vi "CSDB_Transfer.get instance data.vi"(0 "connection reference":T1, 1 "InstanceName":string, 2 "error in (no error)":errorcluster) -> (3 "connection reference out":T1, 4 "InstanceName      Classname":string[](array[string]), 5 "InstanceName      AttributeName      Value":string[][](array[string]), 6 "error out":errorcluster)   [LabVIEW 2014, in "CSDB_Transfer.lvlib"]
uses:
  CSDB_Transfer.lvlib
  <vilib>/addons/database/Connection.llb/Conn ObjectReference.ctl
  <vilib>/addons/database/NI_Database_API.lvlib
  CSDB_Common/CSDB_Common.lvlib
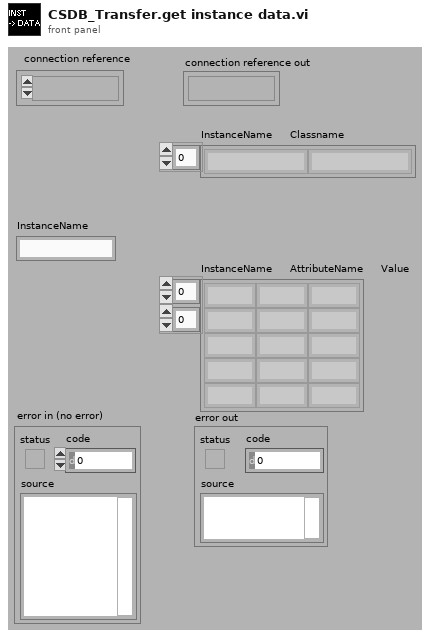
[diagram p1: front panel]
types:
  T1 = typedef "NI_Database_API.lvlib/Conn ObjectReference.ctl" = refnum<k1>
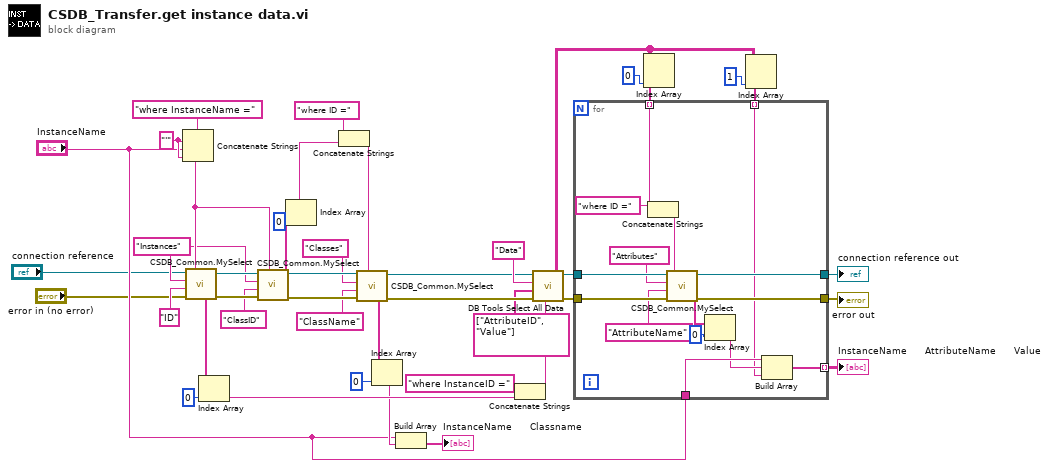
[diagram p0: block diagram]
diagram:
  w37 = "Instances" ("table")
  w42 = "'"
  n1 = Concatenate Strings("where InstanceName =", w42, "InstanceName", w42) -> (w40:string)
  n2 = call "CSDB_Common.MySelect.vi"("optional clause"=w40, "error in (no error)"="error in (no error)", "column"="ID", "table"=w37, "connection reference"="connection reference") -> ("error out"=w38:errorcluster, "1d output array"=w35:string[], "connection reference out"=w39:T1)  [unwired: 2 in]
  n3 = Index Array(array=w35, index=0) -> (element=w15:string)
  n4 = call "CSDB_Common.MySelect.vi"("optional clause"=w40, "error in (no error)"=w38, "column"="ClassID", "table"=w37, "connection reference"=w39) -> ("error out"=w33:errorcluster, "1d output array"=w30:string[], "connection reference out"=w34:T1)  [unwired: 2 in]
  n5 = Index Array(array=w30, index=0) -> (element=w14:string)
  n6 = Concatenate Strings("where ID =", w14) -> (w27:string)
  n7 = call "CSDB_Common.MySelect.vi"("optional clause"=w27, "error in (no error)"=w33, "column"="ClassName", "table"="Classes", "connection reference"=w34) -> ("error out"=w26:errorcluster, "1d output array"=w20:string[], "connection reference out"=w16:T1)  [unwired: 2 in]
  n8 = Index Array(array=w20, index=0) -> (element=w8:string)
  n9 = Build Array("InstanceName", w8) -> (→"InstanceName      Classname":string[])
  n10 = Concatenate Strings("where InstanceID =" ("string"), w15) -> (w22:string)
  n11 = call <vilib>:"DB Tools Select All Data.vi"("optional clause"=w22, "error in (no error)"=w26, "columns"=string[] ["AttributeID", "Value"], "table"="Data", "connection reference"=w16) -> ("error out"=w17:errorcluster, "data"=w13:string[][], "connection reference out"=w18:T1)  [unwired: 1 in]
  n12 = Index Array(array=w13, index (col)=0 ("index")) -> (element=w12:string[])  [unwired: 1 in]
  n13 = Index Array(array=w13, index (col)=1 ("index")) -> (element=w9:string[])  [unwired: 1 in]
  n14 = for {
    tunnel: w18 -> [w58]
    tunnel: w17 -> [w57]
    tunnel: [w51] -> w2
    tunnel: [w50] -> w1
    tunnel: "InstanceName" -> [w49]
    tunnel: [w47] -> w5 mode=indexing
    tunnel: w12 -> [w45] mode=indexing
    tunnel: w9 -> [w44] mode=indexing
    n15 = Concatenate Strings("where ID =" ("string"), w45) -> (w53:string)
    n16 = call "CSDB_Common.MySelect.vi"("optional clause"=w53, "error in (no error)"=w57, "column"="AttributeName", "table"="Attributes", "connection reference"=w58) -> ("error out"=w50:errorcluster, "1d output array"=w52:string[], "connection reference out"=w51:T1)  [unwired: 2 in]
    n17 = Index Array(array=w52, index=0) -> (element=w48:string)
    n18 = Build Array(w49, w48, w44) -> (w47:string[])
  }
  "InstanceName      AttributeName      Value" <- w5
  "connection reference out" <- w2
  "error out" <- w1
